vi "CRYO_FDS_LS218.vi"() -> ()   [LabVIEW 2016]
uses:
  Commande 1.ctl
panel:
  out "NOM_MANIP":string
  out "PERIODE":i8
  out "table_acq":T1(array[cluster])
  out "Celsius":bool
  out "Voies_LS218":T2(array[cluster])
  out "T1_4":i32
  out "T5_8":i32
  out "DOSSIER":path
  out "sortie d'erreur":errorcluster
  in  "entrée d'erreur":errorcluster
  in  "Port_COM":refnum<visa-resource-name>
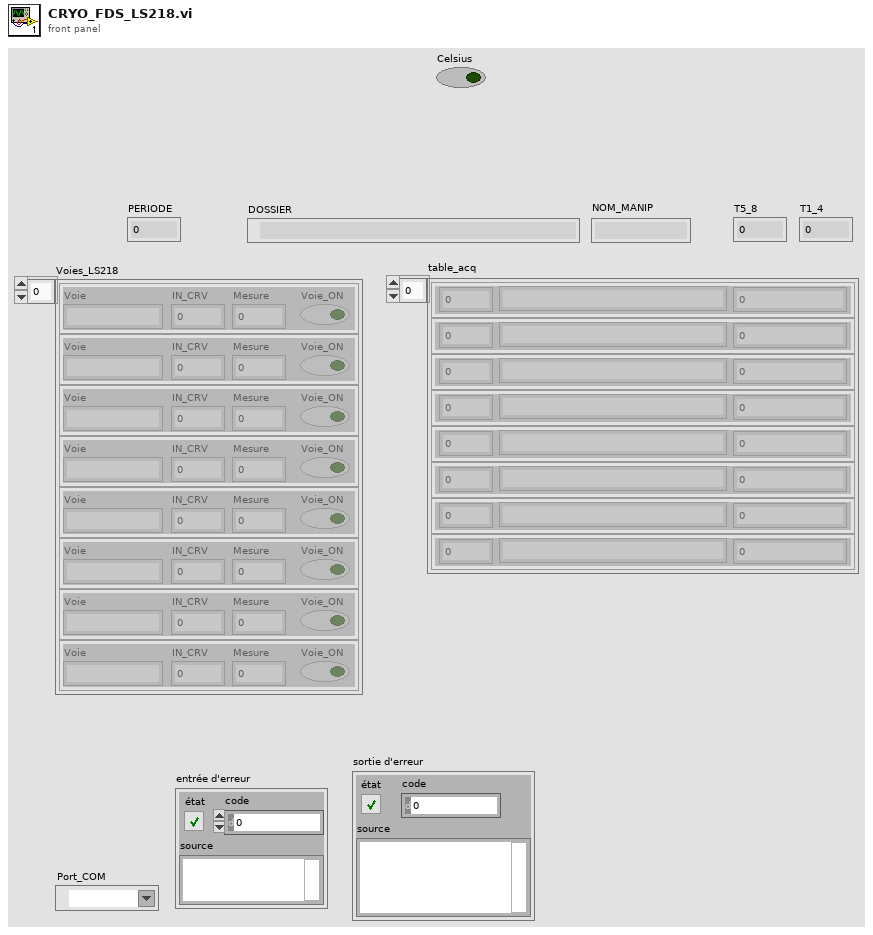
[diagram p1: front panel]
types:
  T1 = cluster{"N_voie":i32, "Nom_voie":string, "Mesure_voie":dbl}[]
  T2 = cluster{"Voie":string, "IN_CRV":u16, "Mesure":dbl, "Voie_ON":bool}[]
  T3 = cluster{"Chaîne":string, "Input_type":u16, "Numérique":dbl, "Booléen":bool}[]
  T4 = typedef "Commande 1.ctl" = enum16{"init", "config", "data", "toto", "erreur", "fin"}
  T5 = enum32{"Invalid", "Standard", "Closed", "Hidden", "Minimized", "Maximized"}
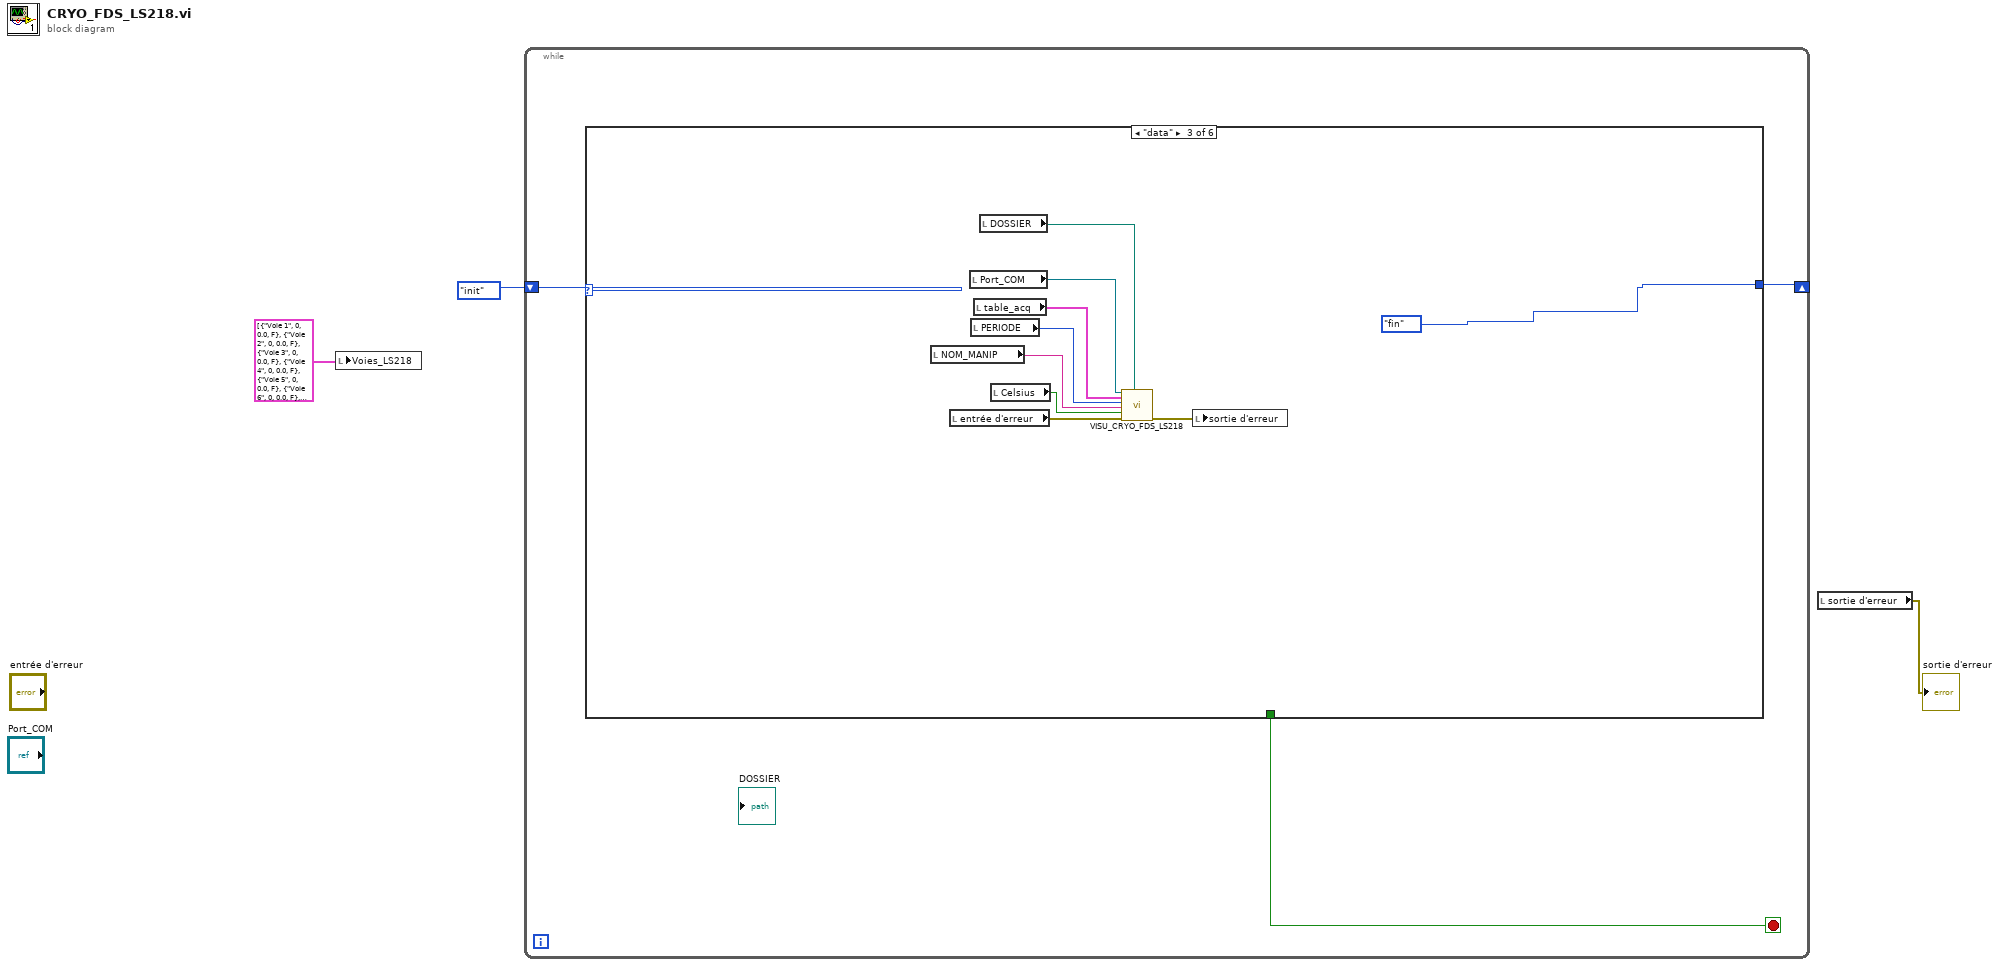
[diagram p0: block diagram]
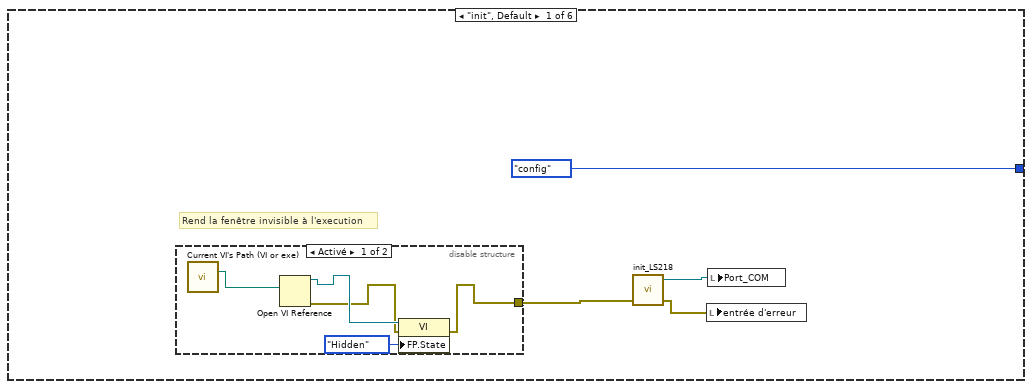
[diagram p2: hidden frame]
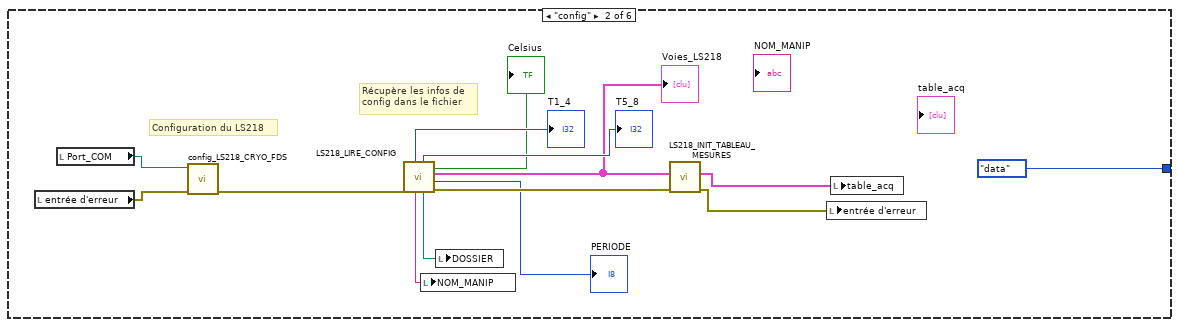
[diagram p4: hidden frame]
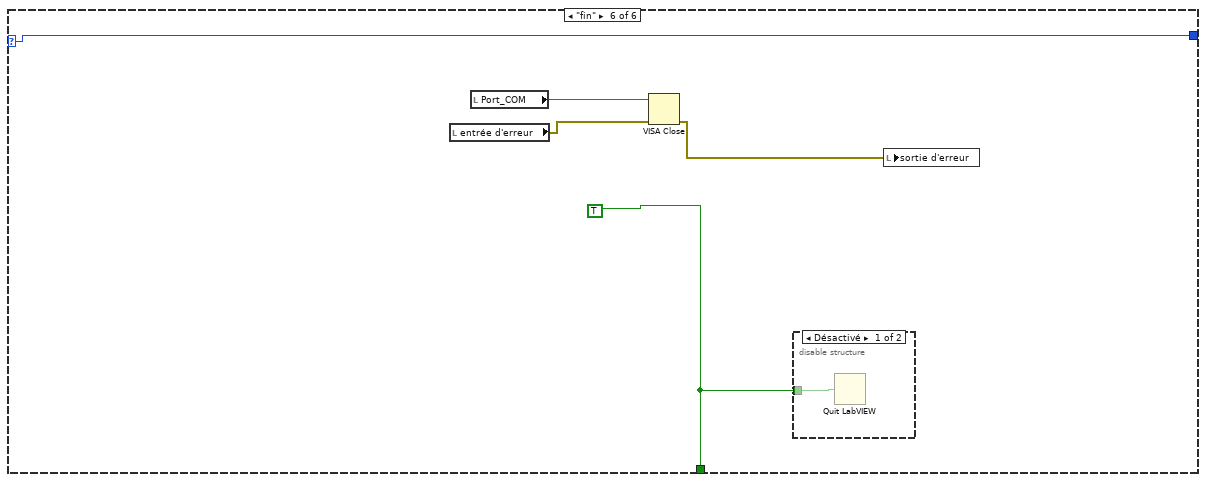
[diagram p7: hidden frame]
diagram:
  n1 = local write "Voies_LS218"(T3 [{"Chaîne"="Voie 1", "Input_type"=0, "Numérique"=0.0, "Booléen"=FALSE}, {"Chaîne"="Voie 2", "Input_type"=0, "Numérique"=0.0, "Booléen"=FALSE}, {"Chaîne"="Voie 3", "Input_type"=0, "Numérique"=0.0, "Booléen"=FALSE}, {"Chaîne"="Voie 4", "Input_type"=0, "Numérique"=0.0, "Booléen"=FALSE}, {"Chaîne"="Voie 5", "Input_type"=0, "Numérique"=0.0, "Booléen"=FALSE}, {"Chaîne"="Voie 6", "Input_type"=0, "Numérique"=0.0, "Booléen"=FALSE}, {"Chaîne"="Voie 7", "Input_type"=0, "Numérique"=0.0, "Booléen"=FALSE}, {"Chaîne"="Voie 8", "Input_type"=0, "Numérique"=0.0, "Booléen"=FALSE}] ("Voies de mesures")) -> ()
  n2 = while {
    shift-right: [w5] -> _
    shift-left: Commande_1."init" ("Énum") -> [w6]
    stop <- w4 stop-if-true
    n3 = case shown="\"data\"" w6 {
      selector: w6 -> [_ _ _ w39 w40 w45]
      tunnel: [Commande_1."config" ("Énum") Commande_1."data" ("Énum") Commande_1."fin" ("cas faux") w39 w40 w45] -> w5
      tunnel: [_ _ _ _ _ w41] -> w4
      frame "init", Default {
        # "Rend la fenêtre invisible à l'execution"
        n4 = disable-structure shown="Activé" {
          disable-tunnel: [w11 _] -> w7
          frame Enabled {
            n5 = call "Current VI's Path (VI or exe).vi"() -> ("Full Path to VI or executable"=w15:path)  [unwired: 14 in, 1 out]
            n6 = Open VI Reference(vi path=w15) -> (vi reference=w14:refnum<vi>, error out=w12:errorcluster)  [unwired: 5 in]
            n7 = property class="VI"(reference=w14, error in=w12, "FP.State"=T5."Hidden" ("Fenêtre face-avant:État")) -> (error out=w11:errorcluster)  [unwired: 1 out]
          }
          frame Disabled {
          }
        }
        n8 = call "init_LS218.vi"("entrée d'erreur"=w7) -> ("sortie d'erreur"=w8:errorcluster, "Nom de ressource VISA en sortie"=w9:refnum<visa-resource-name>)  [unwired: 2 in, 1 out]
        n9 = local write "entrée d'erreur"(w8) -> ()
        n10 = local write "Port_COM"(w9) -> ()
      }
      frame "config" {
        # "Configuration du LS218"
        # "Récupère les infos de \nconfig dans le fichier"
        n11 = local read "entrée d'erreur"() -> (w28:errorcluster)
        n12 = local read "Port_COM"() -> (w20:refnum<visa-resource-name>)
        n13 = call "config_LS218_CRYO_FDS.vi"("entrée d'erreur"=w28, "Port_COM"=w20) -> ("sortie d'erreur"=w27:errorcluster)  [unwired: 9 in]
        n14 = call "LS218_LIRE_CONFIG.vi"("entrée d'erreur (pas d'erreur)"=w27) -> ("sortie d'erreur"=w21:errorcluster, "PERIODE"=→"PERIODE":i8, "Voies de mesures"=w22:T3, "Celsius"=→"Celsius":bool, "DOSSIER"=w26:path, "value 2"=→"T5_8":i32, "NOM MANIP"=w16:string, "value"=→"T1_4":i32)  [unwired: 3 in]
        "Voies_LS218" <- w22
        n15 = local write "NOM_MANIP"(w16) -> ()
        n16 = local write "DOSSIER"(w26) -> ()
        n17 = call "LS218_INIT_TABLEAU_MESURES.vi"("error in (no error)"=w21, "Voies de mesures"=w22) -> ("error out"=w19:errorcluster, "table_acq"=w18:T1)  [unwired: 8 in]
        n18 = local write "entrée d'erreur"(w19) -> ()
        n19 = local write "table_acq"(w18) -> ()
      }
      frame "data" {
        n20 = local read "NOM_MANIP"() -> (w34:string)
        n21 = local read "entrée d'erreur"() -> (w36:errorcluster)
        n22 = local read "Port_COM"() -> (w31:refnum<visa-resource-name>)
        n23 = local read "PERIODE"() -> (w33:i8)
        n24 = local read "table_acq"() -> (w32:T1)
        n25 = local read "DOSSIER"() -> (w30:path)
        n26 = local read "Celsius"() -> (w35:bool)
        n27 = call "VISU_CRYO_FDS_LS218.vi"("Port_COM"=w31, "table_acq"=w32, "PÉRIODE ACQUISITION (sec)"=w33, "Nom manip"=w34, "Celsius?"=w35, "error in (no error)"=w36, "Répertoire"=w30) -> ("error out"=w37:errorcluster)  [unwired: 11 in, 1 out]
        n28 = local write "sortie d'erreur"(w37) -> ()
      }
      frame "toto" {
      }
      frame "erreur" {
      }
      frame "fin" {
        w41 = TRUE ("stop")
        n29 = local read "entrée d'erreur"() -> (w43:errorcluster)
        n30 = local read "Port_COM"() -> (w44:refnum<visa-resource-name>)
        n31 = VISA Close(VISA resource name=w44, error in (no error)=w43) -> (error out=w42:errorcluster)
        n32 = disable-structure shown="Désactivé" {
          disable-tunnel: w41 -> [w46 _]
          frame Disabled {
            n33 = Quit LabVIEW(quit? (T)=w46) -> ()
          }
          frame Enabled {
          }
        }
        n34 = local write "sortie d'erreur"(w42) -> ()
      }
    }
  }
  n35 = local read "sortie d'erreur"() -> (→"sortie d'erreur":errorcluster)
